vi "Global 1.vi"() -> ()   [LabVIEW 2018]
panel:
  out "Boolean":bool
  in  "String":string
  in  "Numeric":dbl
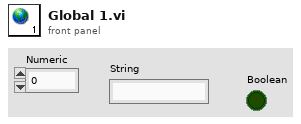
[diagram p1: front panel]
diagram:
